vi "Test Unicode Path UTF8.vi"(8 "error in (no error)":errorcluster) -> (0 "error out":errorcluster, 3 "Pass?":bool)   [LabVIEW 2020]
uses:
  24cb2b3e-0684-4880-b0e7-7c6c3d026634.vi
  G-Audio/Private/Result To Error.vi
  24cb2b3e-0684-4880-b0e7-7c6c3d026634.vi/15efb94c-0eeb-49fd-9ff3-8ea0cffaf39a.vi
  <vilib>/Utility/error.llb/Error Cluster From Error Code.vi
  G-Audio/Private/Copy Data.vi
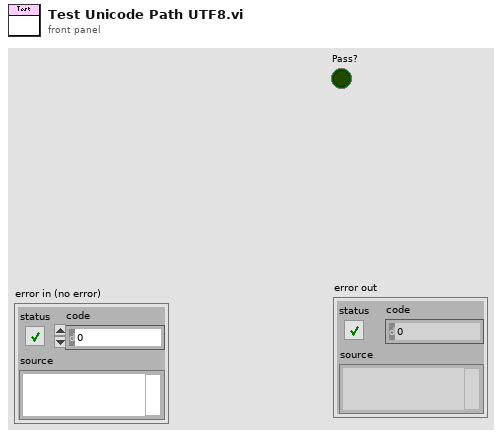
[diagram p1: front panel]
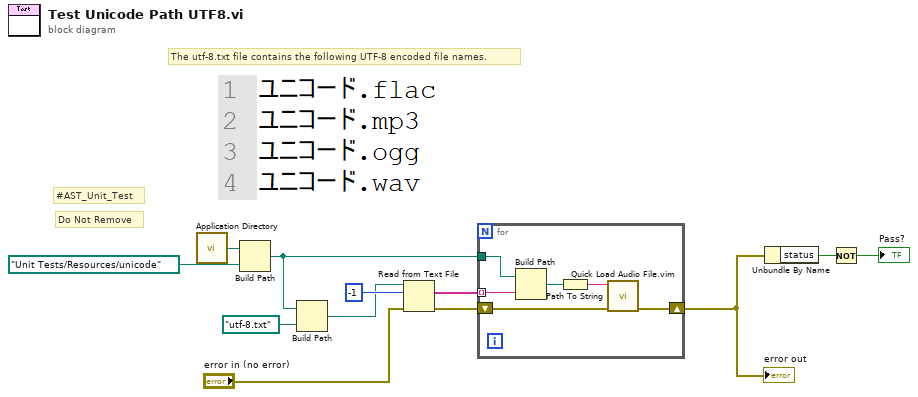
[diagram p0: block diagram]
diagram:
  # "The utf-8.txt file contains the following UTF-8 encoded file names."
  # "Do Not Remove"
  # "#AST_Unit_Test"
  n1 = call <vilib>:"Application Directory.vi"() -> ("Application Directory"=w12:path)
  n2 = Build Path(base path=w12, name or relative path=path "Unit Tests/Resources/unicode" ("Path")) -> (appended path=w6:path)
  n3 = Build Path(base path=w6, name or relative path=path "utf-8.txt") -> (appended path=w8:path)
  n4 = Read from Text File(file (use dialog)=w8, count=-1 ("count (1)"), error in="error in (no error)") -> (text=w10:string[], error out=w2:errorcluster)  [unwired: 1 in, 2 out]
  n5 = for {
    tunnel: w10 -> [w16] mode=indexing
    tunnel: w6 -> [w18]
    shift-right: [w17] -> w1
    shift-left: w2 -> [w13]
    n6 = Build Path(base path=w18, name or relative path=w16) -> (appended path=w15:path)
    n7 = Path To String(path=w15) -> (string=w14:string)
    n8 = call "Quick Load Audio File.vim"("error in (no error)"=w13, "Path"=w14) -> ("error out"=w17:errorcluster)  [unwired: 4 in, 5 out]
  }
  "error out" <- w1
  n9 = Unbundle By Name(w1) -> ("status"=w5:bool)
  n10 = Not(x=w5) -> (.not. x?=→"Pass?":bool)
